vi "Set Image Flip.vi"(10 "iVFlip":i32, 11 "iHFlip":i32) -> (3 "function return":u32)   [LabVIEW 2018, in "Copy of Andor SDK.lvlib"]
doc: "EXPNETTYPE unsigned int WINAPI SetImageFlip(int iHFlip, int iVFlip);"
uses:
  Copy of Andor SDK.lvlib
  <userlib>/Andor SDK/ATMCD32D.dll
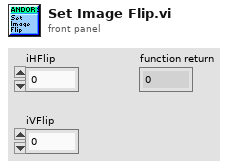
[diagram p1: front panel]
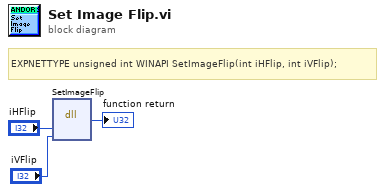
[diagram p0: block diagram]
diagram:
  # "EXPNETTYPE unsigned int WINAPI SetImageFlip(int iHFlip, int iVFlip);"
  n1 = dll-call lib="C:/Program Files (x86)/National Instruments/LabVIEW 2018/user.lib/Andor SDK/ATMCD32D.*" fn="SetImageFlip"("iHFlip"="iHFlip", "iVFlip"="iVFlip") -> (→"function return":u32)  [unwired: 5 in, 2 out]
